vi "Initialize-object.vi"(8 "error in (no error)":errorcluster, 10 "Settings":T1) -> (0 "error out":errorcluster, 3 "Errors out":T3)   [LabVIEW 2013, in "Error-handling.lvlib" / "Errors.lvclass"]
uses:
  Errors.lvclass
  Object-reference.ctl
  Settings.ctl
  Languages.ctl
  Errors.lvclass/Errors.ctl
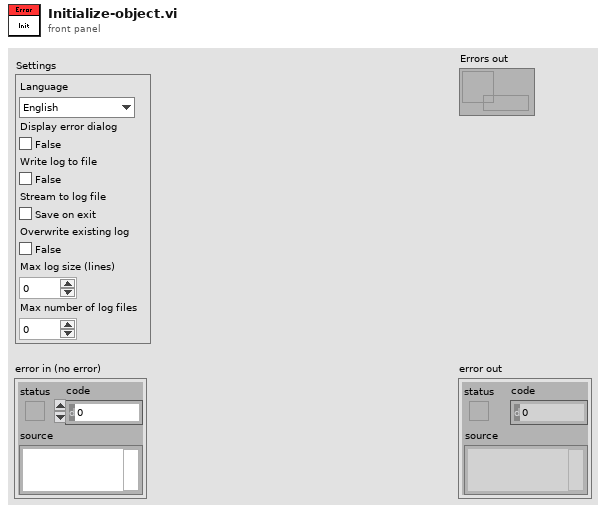
[diagram p1: front panel]
types:
  T1 = typedef "Error-handling.lvlib/Errors.lvclass/Settings.ctl" = cluster{"Language":T2, "Display error dialog":bool, "Write log to file":bool, "Stream to log file":bool, "Overwrite existing log":bool, "Max log size":i32, "Max number of log files":i32}
  T2 = typedef "Error-handling.lvlib/Errors.lvclass/Languages.ctl" = enum16{"English"}
  T3 = typedef "Error-handling.lvlib/Errors.lvclass/Object-reference.ctl" = refnum<data-value>
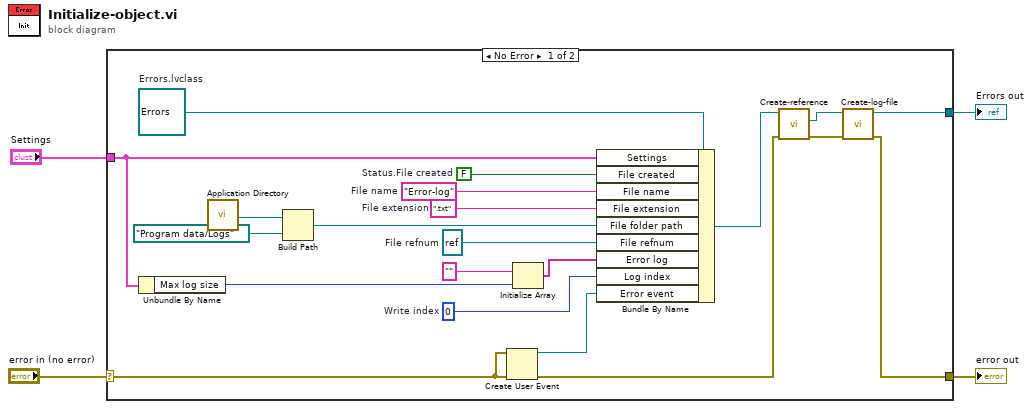
[diagram p0: block diagram]
diagram:
  n1 = case shown="No Error" "error in (no error)" {
    selector: "error in (no error)" -> [w5 w26]
    tunnel: [w13 w26] -> w3
    tunnel: [w12 _] -> w2
    tunnel: "Settings" -> [w9 _]
    frame No Error {
      w10 = FALSE  # Status.File created
      w11 = refnum<class "Errors.lvclass"> refnum  # Errors.lvclass
      w17 = 0  # Write index
      w20 = refnum<file> refnum  # File refnum
      w24 = ".txt"  # File extension
      w25 = "Error-log"  # File name
      n2 = Unbundle By Name(w9) -> ("Max log size"=w8:i32)
      n3 = call <vilib>:"Application Directory.vi"() -> ("Application Directory"=w23:path)
      n4 = Build Path(base path=w23, name or relative path=path "Program data/Logs") -> (appended path=w21:path)
      n5 = Create User Event(user event datatype=w5, error in=w5) -> (user event=w6:refnum<user-event>, error out=w7:errorcluster)
      n6 = Initialize Array("", w8) -> (w19:string[])
      n7 = Bundle By Name(cluster=w11, "Settings"=w9, "File created"=w10, "File name"=w25, "File extension"=w24, "File folder path"=w21, "File refnum"=w20, "Error log"=w19, "Log index"=w17, "Error event"=w6) -> (w16:refnum<class "Errors.lvclass">)
      n8 = call "Create-reference.vi"("error in (no error)"=w7, "Errors in"=w16) -> ("error out"=w14:errorcluster, "Errors reference"=w15:T3)  [unwired: 7 in, 1 out]
      n9 = call "Create-log-file.vi"("error in (no error)"=w14, "Errors in"=w15) -> ("error out"=w13:errorcluster, "Errors out"=w12:T3)  [unwired: 8 in]
    }
    frame Error {
    }
  }
  "error out" <- w3
  "Errors out" <- w2
